vi "Nested Exist.vi"(11 "jettl in":refnum<class "jettl.lvclass">) -> (2 "Nested Exist?":bool)   [LabVIEW 2021, in "jettl.lvlib" / "jettl.lvclass"]
uses:
  jettl.lvclass
  jettl.lvclass/jettl.ctl
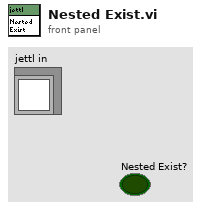
[diagram p1: front panel]
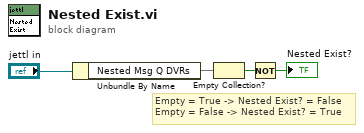
[diagram p0: block diagram]
diagram:
  # "Empty = True -> Nested Exist? = False\nEmpty = False -> Nested Exist? = True"
  n1 = Unbundle By Name("jettl in") -> ("Nested Msg Q DVRs"=w2:set{refnum<data-value>})
  n2 = Empty Collection?(1:w2) -> (0:w4:bool)
  n3 = Not(x=w4) -> (.not. x?=→"Nested Exist?":bool)
